vi "Set Physical Channels.vi"(7 "Channels":i32=16, 10 "signal type":string, 11 "Board Description":string) -> (3 "String":string)   [LabVIEW 2018]
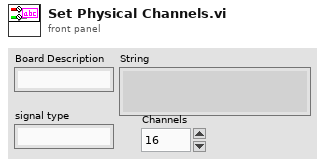
[diagram p1: front panel]
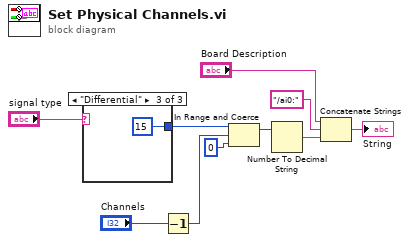
[diagram p0: block diagram]
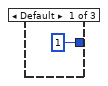
[diagram p2: hidden frame]
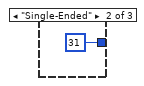
[diagram p3: hidden frame]
diagram:
  n1 = case shown="\"Differential\"" "signal type" {
    tunnel: [1 ("lower limit") 31 ("lower limit") 15 ("lower limit")] -> w3
    frame Default {
    }
    frame "Single-Ended" {
    }
    frame "Differential" {
    }
  }
  n2 = Decrement(x="Channels") -> (x-1=w4:i32)
  n3 = In Range and Coerce(upper limit=w3, x=w4, lower limit=0) -> (coerced(x)=w2:i32)  [unwired: 1 out]
  n4 = Number To Decimal String(number=w2) -> (decimal integer string=w1:string)  [unwired: 1 in]
  n5 = Concatenate Strings("Board Description", "/ai0:" ("string"), w1) -> (→"String":string)
